vi "nanocal-frontend-tcplink-client -- V2.vi"() -> ()   [LabVIEW 2020]
doc: "Demonstrates how to open a connection to an TCP server, read the data being sent, and display the data on a chart. This VI is designed to stop if the TCP connection is terminated."
uses:
  nanocal server folder LV18/icicle.ctl
  publisher action.ctl
panel:
  in  "Server Closed":string="The server VI closed the connection."
  in  "Tab Control":enum32{"Page 1", "Page 2"}(tab)
  in  "Stop":bool
  in  "address":string="146.201.231.45"
  in  "port":u16=6340
  in  "wait (ms)":u32=100
  out "nanocal data array OUT":T1[](array[typedef])
  # "nanocal tcplink --- client"
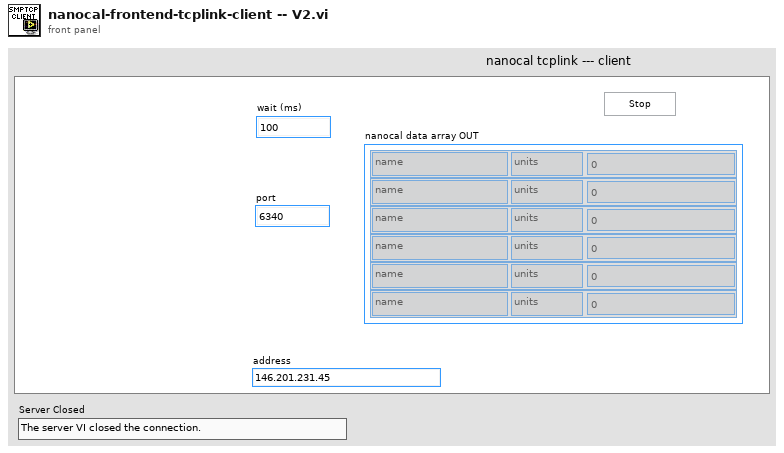
[diagram p1: front panel]
types:
  T1 = typedef "icicle.ctl" = cluster{"name":string, "units":string, "data":dbl}
  T2 = typedef "publisher action.ctl" = enum16{"set", "get", "init", "check"}
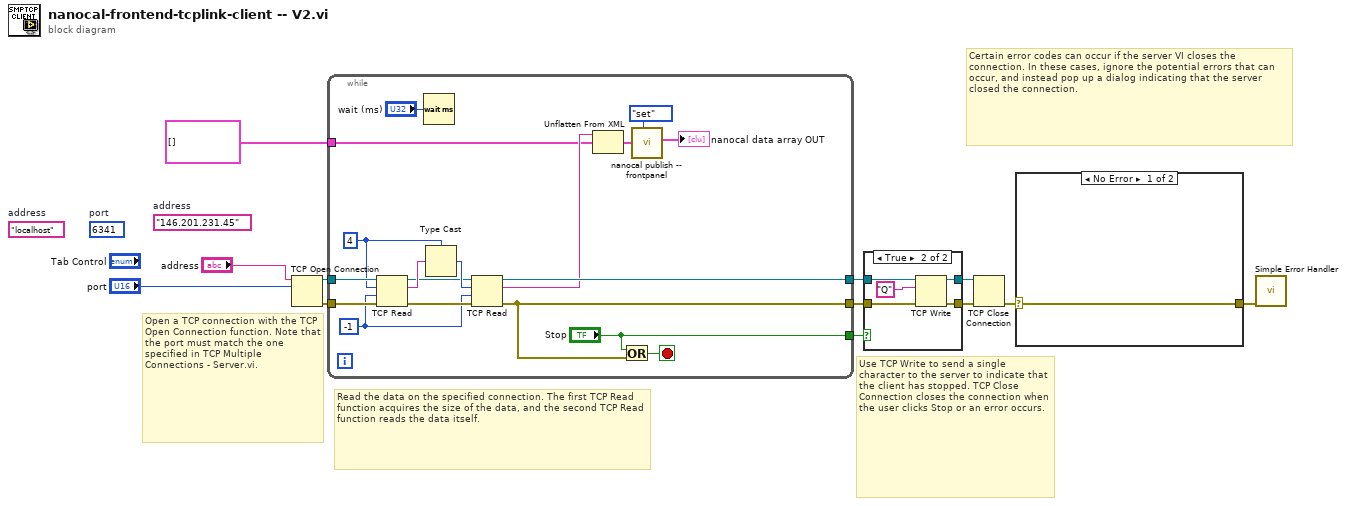
[diagram p0: block diagram]
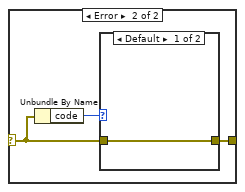
[diagram p2: hidden frame]
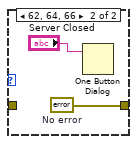
[diagram p3: hidden frame]
diagram:
  (unwired) u16 6341  # port
  (unwired) "localhost"  # address
  (unwired) "146.201.231.45"  # address
  # "Certain error codes can occur if the server VI closes the connection. In these cases, ignore the potential errors that can occur, and instead pop up a dialog indicating that the server closed the connection."
  # "Use TCP Write to send a single character to the server to indicate that the client has stopped. TCP Close Connection closes the connection when the user clicks Stop or an error occurs."
  # "Read the data on the specified connection. The first TCP Read function acquires the size of the data, and the second TCP Read function reads the data itself."
  # "Open a TCP connection with the TCP Open Connection function. Note that the port must match the one specified in TCP Multiple Connections - Server.vi."
  n1 = TCP Open Connection(address="address", remote port or service name="port") -> (connection ID=w12:refnum<k5>, error out=w11:errorcluster)  [unwired: 1 in, 2 out]
  n2 = while {
    tunnel: ["Stop"] -> w6
    tunnel: [w24] -> w10
    tunnel: [w22] -> w8
    tunnel: w11 -> [w29]
    tunnel: w12 -> [w30]
    tunnel: T1[] [] -> [w13]
    stop <- w23 stop-if-true
    w20 = -1
    w21 = 4
    n3 = TCP Read(connection ID=w30, bytes to read=w21, error in (no error)=w29, 9:w20) -> (connection ID out=w25:refnum<k5>, data out=w28:string, error out=w27:errorcluster)  [unwired: 1 out]
    n4 = Wait (ms)(milliseconds to wait="wait (ms)") -> ()  [unwired: 1 out]
    n5 = Type Cast(type=w21, x=w28) -> (*(type *) &x=w26:i32)
    n6 = TCP Read(connection ID=w25, bytes to read=w26, error in (no error)=w27, 9:w20) -> (connection ID out=w24:refnum<k5>, data out=w16:string, error out=w22:errorcluster)  [unwired: 1 out]
    n7 = Unflatten From XML(xml string=w16, type=w13) -> (value=w18:T1[])  [unwired: 1 in, 1 out]
    n8 = Or(x="Stop", y=w22) -> (x .or. y?=w23:bool)
    n9 = call "nanocal publish -- frontpanel.vi"("publisher action"=publisher_action."set", "nanocal data array IN"=w18) -> ("nanocal data array OUT"=→"nanocal data array OUT":T1[])  [unwired: 9 in]
  }
  n10 = case shown="True" w6 {
    tunnel: w10 -> [w32 w37]
    tunnel: [w32 w35] -> w9
    tunnel: w8 -> [w31 w36]
    tunnel: [w31 w34] -> w7
    frame False {
    }
    frame True {
      n11 = TCP Write(connection ID=w37, data in="Q", error in (no error)=w36) -> (connection ID out=w35:refnum<k5>, error out=w34:errorcluster)  [unwired: 2 out]
    }
  }
  n12 = TCP Close Connection(connection ID=w9, error in (no error)=w7) -> (error out=w5:errorcluster)  [unwired: 2 out]
  n13 = case shown="No Error" w5 {
    selector: w5 -> [w38 w40]
    tunnel: [w38 w39] -> w4
    frame No Error {
    }
    frame Error {
      n14 = Unbundle By Name(w40) -> ("code"=w41:i32)
      n15 = case shown="Default" w41 {
        tunnel: w40 -> [w42 _]
        tunnel: [w42 w44] -> w39
        frame Default {
        }
        frame 62, 64, 66 {
          w44 = errorcluster {"status"=FALSE, "code"=0, "source"=""}  # No error
          n16 = One Button Dialog(message="Server Closed") -> ()  [unwired: 1 in, 1 out]
        }
      }
    }
  }
  n17 = call <vilib>:"Simple Error Handler.vi"("error in (no error)"=w4) -> ()  [unwired: 1 in, 8 out]
